vi "MGI Get VI Control Ref[] - backup.vi"(8 "error in":errorcluster, 9 "Include Tab Page Controls? (T)":bool=TRUE, 11 "VI (Caller)":refnum<vi>) -> (0 "error out":errorcluster, 1 "Control Type[i]":T1[](array[typedef]), 2 "Control Label Chain[i]":string[](array[string]), 3 "Control[i]":refnum<vi>[](array[refnum]))   [LabVIEW 2020]
doc: "Returns refnums of all controls on a front panel. If <B>Include Tab Page Controls</B> is true, then all controls on tab pages are included recursively.\nThe type of each returned refnum is also output in <B>Control Type[i]</B>. <B>Control Label[i]</B> contains the label of each control.\n\nAuthored by Martin Weiss, Shawn Walpole\nsupport@mooregoodideas.com\nwww.mooregoodideas.com\n\nCopyright (c) 2010, Moore Good Ideas, Inc.\n\nAll rights reserved.\n\nRedistribution and use in source and binary forms, with or without modification, are permitted provided that the following conditions are met:\n\n * Redistributions of source code must retain the above copyright notice, this list of conditions and the following disclaimer.\n * Redistributions in binary form must reproduce the above copyright notice, this list of conditions and the following disclaimer in the documentation and/or other materials provided with the distribution.\n * Neither the name of Moore Good Ideas, Inc. nor the names of its contributors may be used to endorse or promote products derived from this software without specific prior written permission.\n\nTHIS SOFTWARE IS PROVIDED BY THE COPYRIGHT HOLDERS AND CONTRIBUTORS \"AS IS\" AND ANY EXPRESS OR IMPLIED WARRANTIES, INCLUDING, BUT NOT LIMITED TO, THE IMPLIED WARRANTIES OF MERCHANTABILITY AND FITNESS FOR A PARTICULAR PURPOSE ARE DISCLAIMED. IN NO EVENT SHALL THE COPYRIGHT OWNER OR CONTRIBUTORS BE LIABLE FOR ANY DIRECT, INDIRECT, INCIDENTAL, SPECIAL, EXEMPLARY, OR CONSEQUENTIAL DAMAGES (INCLUDING, BUT NOT LIMITED TO, PROCUREMENT OF SUBSTITUTE GOODS OR SERVICES; LOSS OF USE, DATA, OR PROFITS; OR BUSINESS INTERRUPTION) HOWEVER CAUSED AND ON ANY THEORY OF LIABILITY, WHETHER IN CONTRACT, STRICT LIABILITY, OR TORT (INCLUDING NEGLIGENCE OR OTHERWISE) ARISING IN ANY WAY OUT OF THE USE OF THIS SOFTWARE, EVEN IF ADVISED OF THE POSSIBILITY OF SUCH DAMAGE."
uses:
  <userlib>/_OpenG.lib/appcontrol/appcontrol.llb/ClassID Names Enum__ogtk.ctl
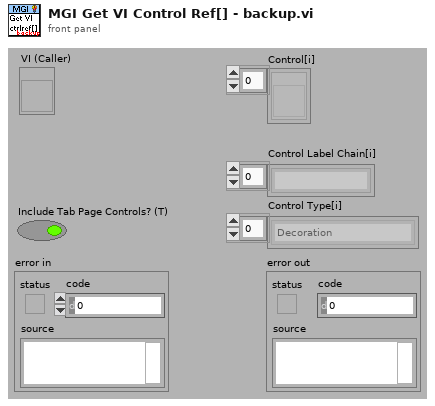
[diagram p1: front panel]
types:
  T1 = typedef "ClassID Names Enum__ogtk.ctl" = enum32{"0 <undefined>", "1 <undefined>", "2 <undefined>", "Generic", "Decoration", "Text", "Control", "ColorBox", "Boolean", "RefNum", "Variant", "Path", "ListBox", "Table", "Array", "Picture", "ActiveXContainer", "Numeric", "Digital", "NamedNumeric", "ColorRamp", "Slide", "GraphOrChart", "WaveformChart", "WaveformGraph", "IntensityChart", "IntensityGraph", "String", "IOName", "ComboBox", "Cluster", "Panel", "Knob", "NumWithScale", "Ring", "Enum", "GObject", "Plot", "Cursor", "NumericText", "Scale", "ColorScale", "GraphScale", "ColorGraphScale", "TypedRefNum", "OldKnobScale", "MCListbox", "MeasureData", "BVTag", "DAQName", "VISAName", "IVIName", "SlideScale", "TabControl", "Page", "TabArrayTabControl", "ConPane"}
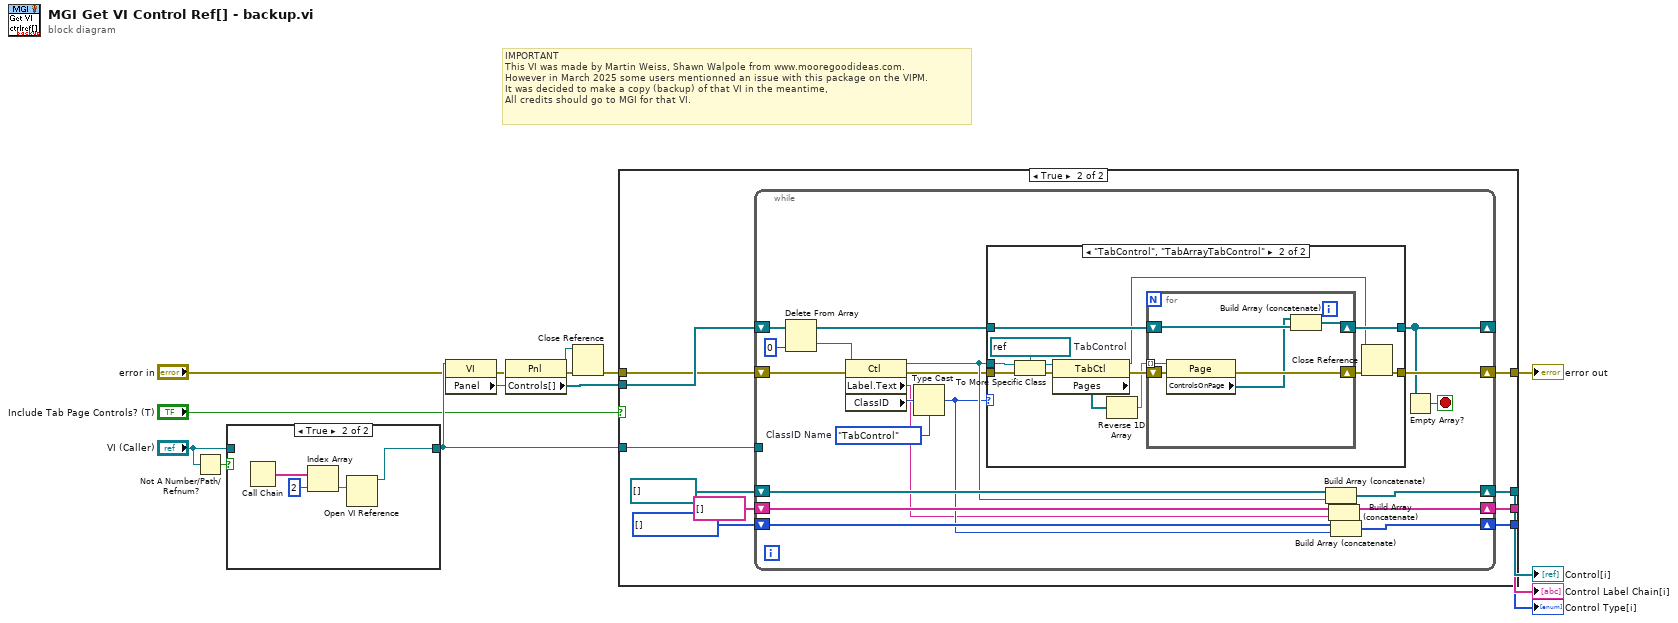
[diagram p0: block diagram]
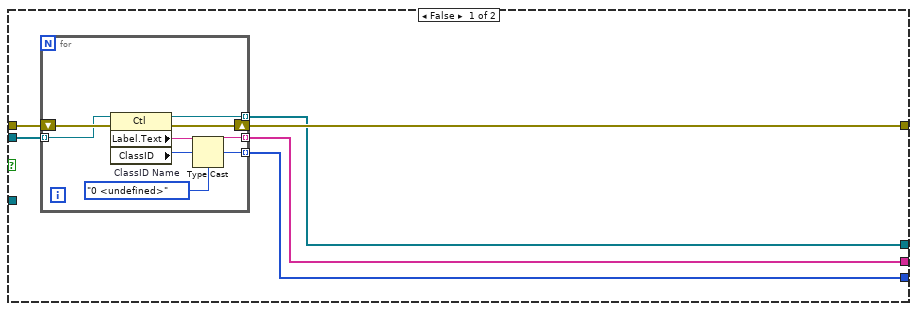
[diagram p2: hidden frame]
diagram:
  # "IMPORTANT\nThis VI was made by Martin Weiss, Shawn Walpole from www.mooregoodideas.com.\nHowever in March 2025 some users mentionned an issue with this package on the VIPM.\nIt was decided to make a copy (backup) of that VI in the meantime,\nAll credits should go to MGI for that VI."
  n1 = Not A Number/Path/Refnum?(number/path/refnum="VI (Caller)") -> (NaN/Path/Refnum?=w13:bool)
  n2 = case shown="True" w13 {
    tunnel: "VI (Caller)" -> [w16 _]
    tunnel: [w16 w20] -> w9
    frame False {
    }
    frame True {
      n3 = Call Chain() -> (call chain=w17:string[])
      n4 = Index Array(array=w17, index=2) -> (element=w18:string)
      n5 = Open VI Reference(vi path=w18) -> (vi reference=w20:refnum<vi>)  [unwired: 5 in, 1 out]
    }
  }
  n6 = property class="VI"(reference=w9, error in="error in") -> (error out=w10:errorcluster, "Panel"=w11:refnum<vi>)  [unwired: 1 out]
  n7 = property class="Pnl"(reference=w11, error in=w10) -> (reference out=w5:refnum<vi>, error out=w7:errorcluster, "Controls[]"=w1:refnum<vi>[])
  n8 = Close Reference(reference=w5, error in (no error)=w7) -> (error out=w6:errorcluster)
  n9 = case shown="True" "Include Tab Page Controls? (T)" {
    tunnel: [w24 w44] -> w15
    tunnel: [w23 w39] -> w14
    tunnel: w9 -> [_ w43]
    tunnel: w1 -> [w26 w42]
    tunnel: w6 -> [w25 w41]
    tunnel: [w22 w37] -> w3
    tunnel: [w21 w36] -> w2
    frame False {
      n10 = for {
        tunnel: w26 -> [w27] mode=indexing
        shift-right: [w34] -> w24
        shift-left: w25 -> [w33]
        tunnel: [w32] -> w22 mode=indexing
        tunnel: [w28] -> w21 mode=indexing
        tunnel: [w31] -> w23 mode=indexing
        w30 = ClassID_Names_Enum__ogtk."0 <undefined>"  # ClassID Name
        n11 = property class="Ctl"(reference=w27, error in=w33) -> (reference out=w31:refnum<vi>, error out=w34:errorcluster, "Label.Text"=w32:string, "ClassID"=w29:u32)
        n12 = Type Cast(type=w30, x=w29) -> (*(type *) &x=w28:T1)
      }
    }
    frame True {
      w35 = T1[] [] items=["0 <undefined>", "1 <undefined>", "2 <undefined>", "Generic", "Decoration", "Text", "Control", "ColorBox", "Boolean", "RefNum", "Variant", "Path", "ListBox", "Table", "Array", "Picture", "ActiveXContainer", "Numeric", "Digital", "NamedNumeric", "ColorRamp", "Slide", "GraphOrChart", "WaveformChart", "WaveformGraph", "IntensityChart", "IntensityGraph", "String", "IOName", "ComboBox", "Cluster", "Panel", "Knob", "NumWithScale", "Ring", "Enum", "GObject", "Plot", "Cursor", "NumericText", "Scale", "ColorScale", "GraphScale", "ColorGraphScale", "TypedRefNum", "OldKnobScale", "MCListbox", "MeasureData", "BVTag", "DAQName", "VISAName", "IVIName", "SlideScale", "TabControl", "Page", "TabArrayTabControl", "ConPane"]
      n13 = while {
        tunnel: w43 -> [_]
        shift-right: [w59] -> _
        shift-left: w42 -> [w63]
        shift-right: [w64] -> w44
        shift-left: w41 -> [w49]
        shift-right: [w57] -> w39
        shift-left: refnum<vi>[] [] -> [w60]
        shift-right: [w53] -> w37
        shift-left: string[] [] -> [w52]
        shift-right: [w51] -> w36
        shift-left: w35 -> [w50]
        stop <- w58 stop-if-true
        w54 = ClassID_Names_Enum__ogtk."TabControl"  # ClassID Name
        n14 = Delete From Array(array=w63, index=0) -> (deleted portion=w46:refnum<vi>, array with subset deleted=w61:refnum<vi>[])  [unwired: 1 in]
        n15 = property class="Ctl"(reference=w46, error in=w49) -> (reference out=w56:refnum<vi>, error out=w48:errorcluster, "Label.Text"=w45:string, "ClassID"=w55:u32)
        n16 = Type Cast(type=w54, x=w55) -> (*(type *) &x=w47:T1)
        n17 = case shown="\"TabControl\", \"TabArrayTabControl\"" w47 {
          tunnel: [w65 w79] -> w64
          tunnel: w61 -> [w66 w78]
          tunnel: [w66 w75] -> w59
          tunnel: w56 -> [_ w74]
          tunnel: w48 -> [w65 w69]
          frame Default {
          }
          frame "TabControl", "TabArrayTabControl" {
            w76 = refnum<vi> refnum  # TabControl
            n18 = To More Specific Class(target class=w76, reference=w74, error in=w69) -> (specific class reference=w77:refnum<vi>, error out=w70:errorcluster)
            n19 = property class="TabCtl"(reference=w77, error in=w70) -> (reference out=w72:refnum<vi>, error out=w73:errorcluster, "Pages"=w68:refnum<vi>[])
            n20 = Reverse 1D Array(array=w68) -> (reversed array=w67:refnum<vi>[])
            n21 = for {
              tunnel: w67 -> [w85] mode=indexing
              shift-right: [w83] -> w71
              shift-left: w73 -> [w84]
              shift-right: [w82] -> w75
              shift-left: w78 -> [w81]
              n22 = property class="Page"(reference=w85, error in=w84) -> (error out=w83:errorcluster, "ControlsOnPage"=w80:refnum<vi>[])  [unwired: 1 out]
              n23 = Build Array (concatenate)(w80, w81) -> (w82:refnum<vi>[])
            }
            n24 = Close Reference(reference=w72, error in (no error)=w71) -> (error out=w79:errorcluster)
          }
        }
        n25 = Build Array (concatenate)(w60, w56) -> (w57:refnum<vi>[])
        n26 = Build Array (concatenate)(w52, w45) -> (w53:string[])
        n27 = Build Array (concatenate)(w50, w47) -> (w51:T1[])
        n28 = Empty Array?(array=w59) -> (empty?=w58:bool)
      }
    }
  }
  "error out" <- w15
  "Control[i]" <- w14
  "Control Type[i]" <- w2
  "Control Label Chain[i]" <- w3
